vi "M3202 generate wave.vi"() -> ()   [LabVIEW 2020]
panel:
  in  "nSlot":i32=3
  in  "nChassis":i32=1
  out "errorOut":errorcluster
  in  "frequency Hz":dbl=10000000.0 format="%^#_6e"
  in  "amplitude V":dbl=0.2
  in  "waveShape":i32(ring)=1 items=["HiZ"=-1, "Off"=0, "Sinusoidal"=1, "Triangular"=2, "Sawtooth"=3, "Square"=4, "DC"=5, "AWG"=6, "Partner"=8]
  in  "nChannel":i32=1
  in  "errorIn":errorcluster
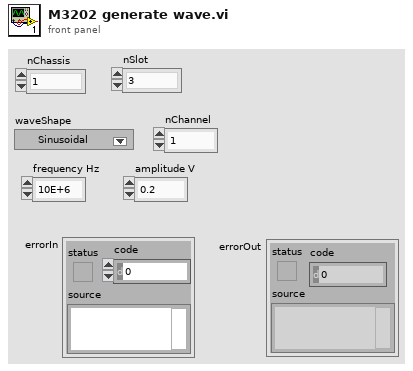
[diagram p1: front panel]
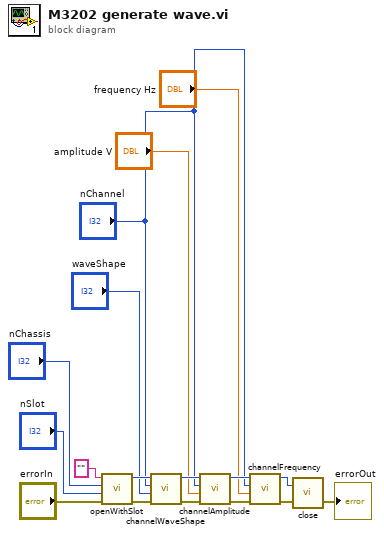
[diagram p0: block diagram]
diagram:
  n1 = call <vilib>:"openWithSlot.vi"("errorIn"="errorIn", "nSlot"="nSlot", "nChassis"="nChassis", "partNumber"="") -> ("errorOut"=w14:errorcluster, "moduleID"=w15:i32)  [unwired: 2 in]
  n2 = call <vilib>:"channelWaveShape.vi"("errorIn"=w14, "waveShape"="waveShape", "nChannel"="nChannel", "moduleID"=w15) -> ("errorOut"=w10:errorcluster, "moduleIDOut"=w12:i32)  [unwired: 2 in]
  n3 = call <vilib>:"channelAmplitude.vi"("errorIn"=w10, "amplitude"="amplitude V", "nChannel"="nChannel", "moduleID"=w12) -> ("errorOut"=w8:errorcluster, "moduleIDOut"=w9:i32)  [unwired: 2 in]
  n4 = call <vilib>:"channelFrequency.vi"("errorIn"=w8, "frequency"="frequency Hz", "nChannel"="nChannel", "moduleID"=w9) -> ("errorOut"=w5:errorcluster, "moduleIDOut"=w4:i32)  [unwired: 2 in]
  n5 = call <vilib>:"close.vi"("errorIn"=w5, "moduleID"=w4) -> ("errorOut"=→"errorOut":errorcluster)  [unwired: 1 in]
